vi "Concatenate URL.vi"(8 "error in (no error)":errorcluster, 10 "Child Name":string, 11 "Parent URL":refnum<k21>) -> (0 "error out":errorcluster, 3 "Child URL":refnum<k21>)   [LabVIEW 2024]
doc: "Builds a child URL from a parent URL and a child name string."
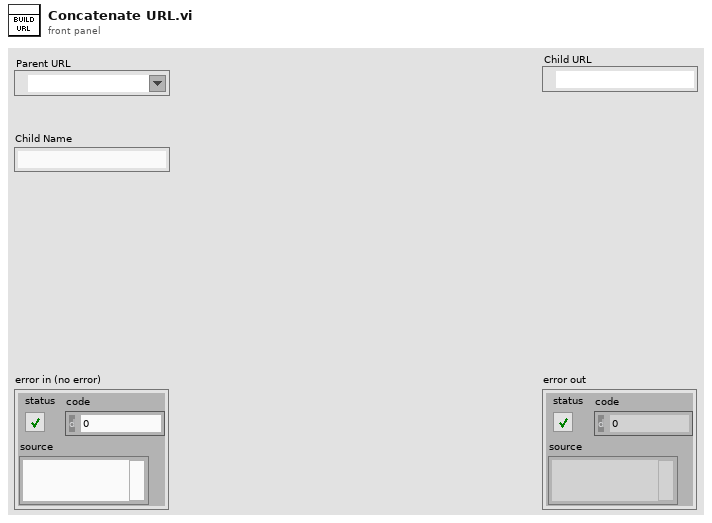
[diagram p1: front panel]
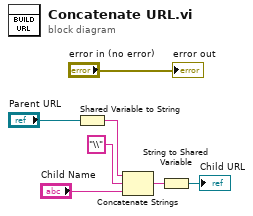
[diagram p0: block diagram]
diagram:
  n1 = Shared Variable to String(1:"Parent URL") -> (0:w2:string)
  n2 = Concatenate Strings(w2, "\\" ("string"), "Child Name") -> (w1:string)
  n3 = String to Shared Variable(0:w1) -> (2:→"Child URL":refnum<k21>)  [unwired: 1 out]
  "error out" <- "error in (no error)"
